vi "Read Genes.vi"(8 "error in (no error)":errorcluster, 11 "IChromosome in":refnum<class "IChromosome.lvclass">) -> (0 "error out":errorcluster, 2 "Genes":refnum<class "IGene.lvclass">[](array[class]), 3 "IChromosome out":refnum<class "IChromosome.lvclass">)   [LabVIEW 2016, in "IChromosome.lvclass"]
uses:
  IChromosome.lvclass
  IGene/IGene.lvclass
  IChromosome.lvclass/IChromosome.ctl
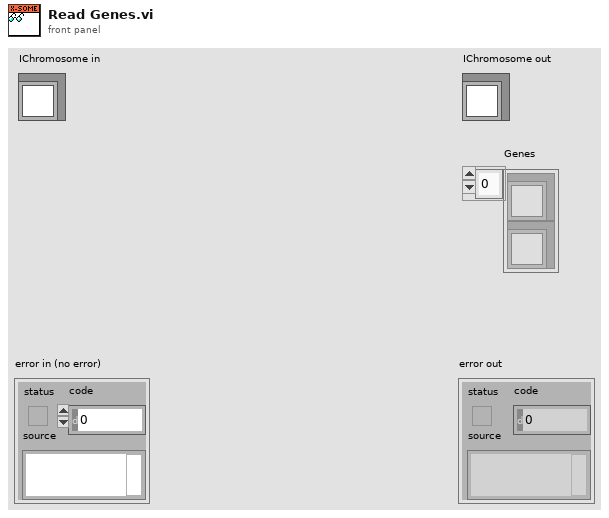
[diagram p1: front panel]
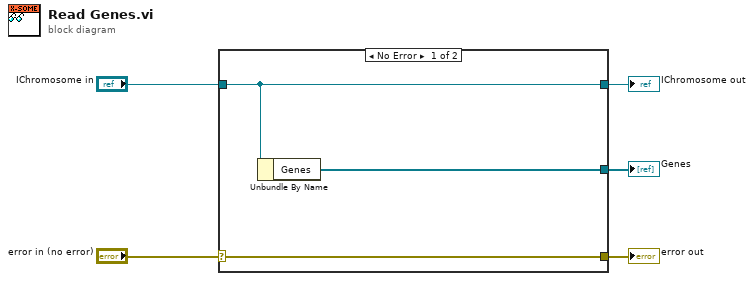
[diagram p0: block diagram]
diagram:
  n1 = case shown="No Error" "error in (no error)" {
    selector: "error in (no error)" -> [w8 w9]
    tunnel: [w8 w9] -> w4
    tunnel: [w7 w10] -> w2
    tunnel: "IChromosome in" -> [w7 w10]
    tunnel: [w6 _] -> w1
    frame No Error {
      n2 = Unbundle By Name(w7) -> ("Genes"=w6:refnum<class "IGene.lvclass">[])
    }
    frame Error {
    }
  }
  "error out" <- w4
  "IChromosome out" <- w2
  "Genes" <- w1
